vi "main_trackVideoFile.vi"() -> ()   [LabVIEW 2013]
uses:
  <vilib>/vision/Image Controls.llb/IMAQ Image.ctl
  <vilib>/vision/Avi.llb/IMAQ AVI2 Refnum.ctl
panel:
  out "Fitted Image":T1
  in  "SessionID":string
  in  "Exit program":bool
  in  "Start Session":bool
  in  "Tab Control":T2(tab)
  out "Eyetracker":T1(plugin-control)
  out "Pupil Radius":dbl[](graph)
  out "Avg freq":dbl caption="Eyetracker - Mean \nprocessing frequency (Hz)" format="%0.2f"
  in  "Save data to disk":bool
  out "Pupil marked":bool=TRUE
  out "Processed":T1(plugin-control)
  in  "Slowmo":bool=TRUE
  in  "Realtime":bool=TRUE
  in  "Fps to save images":u16(ring) items=["30", "60", "90", "120"]
  in  "Camera Fps":u16(ring) items=["30", "60", "90", "120"]
  in  "Look For (Threshold 2)":u32(ring)=1 items=["Bright Objects", "Dark Objects"]
  in  "Start / Stop Tracking":bool
  out "AVI Refnum - Eye":T3
  in  "Manual Threshold":cluster{sgl, sgl}(slide)={0.0, 150.0} caption="Threshold Range" scale=0.0..255.0
  in  "Pupiltracker Cam Connected":bool=TRUE
  out "Cropped Image":T1
  out "Processed Image":T1
  in  "Save folder":path=path "C:/Users/Eivind/Desktop"
  in  "Input video File":path=path "D:/RotationExperiments_v3_GCaMP6f+tdTomato/mouse013/session-m013-20161122-1807/labview_data/Block-11222016-1807-001-LightsON/EyeTracker-11222016-1807-001.avi"
  # "Optimize Tracking"
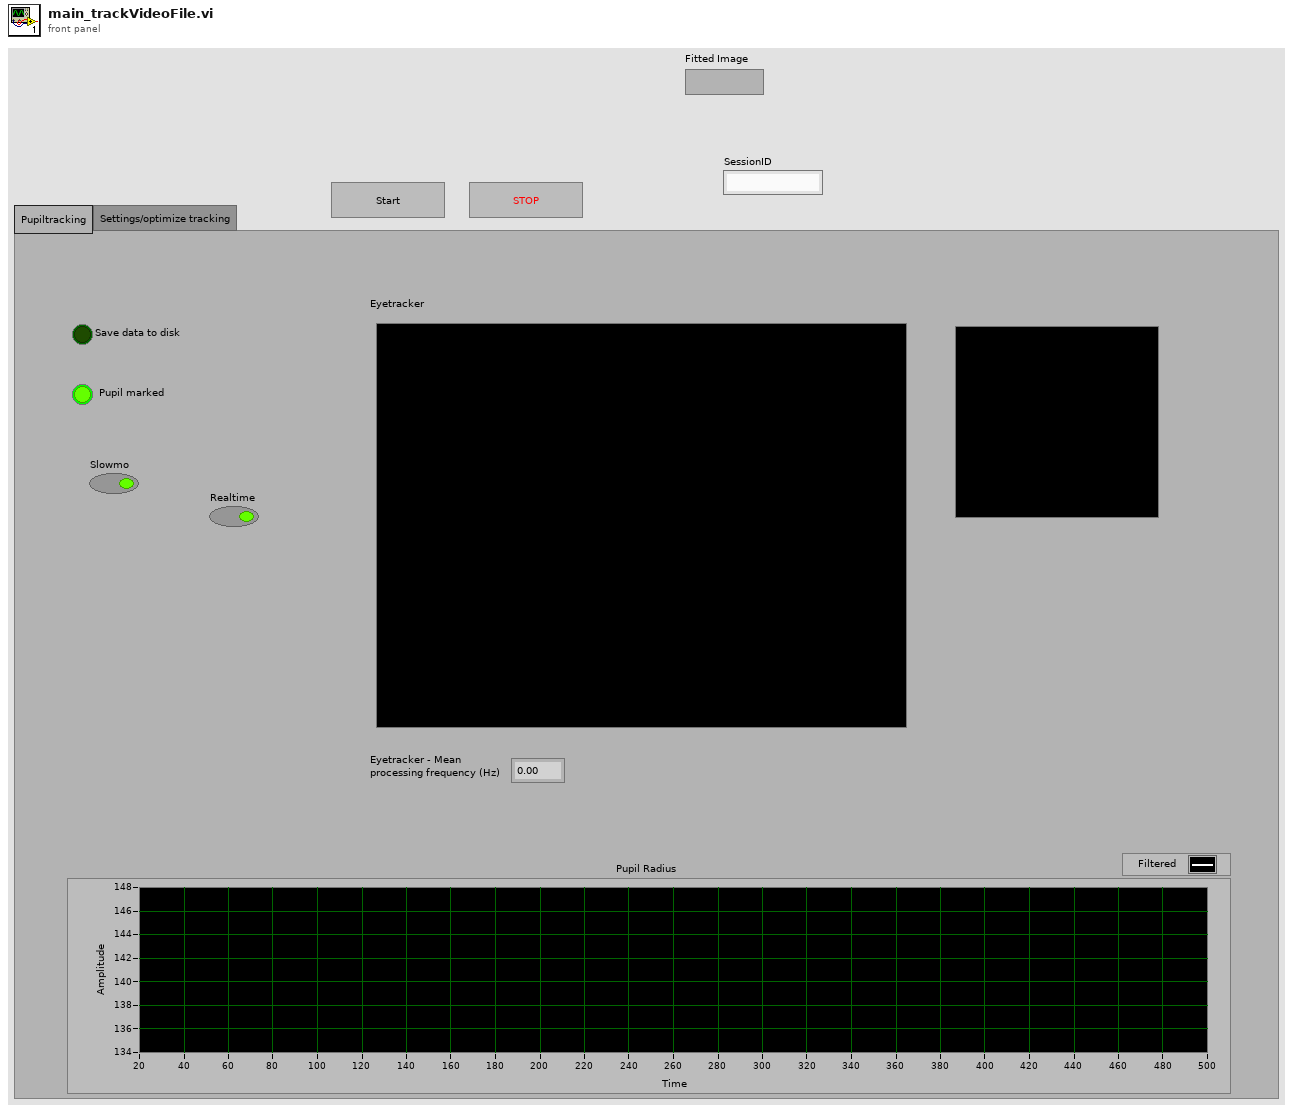
[diagram p1: front panel]
types:
  T1 = typedef "IMAQ Image.ctl" = refnum<image>
  T2 = enum32{"Pupiltracking", "Settings/optimize tracking"}
  T3 = typedef "IMAQ AVI2 Refnum.ctl" = refnum<k20>
  T4 = typedef "Image Type" = u32
  T5 = cluster{"Frame No":i32, "Circle time series":dbl[][], "Rectangle coordinates":i32[], "Annulus ROI":cluster{"ID":enum32{"External", "Internal"}, "Type":u32, i32[]}, "Annulus coordinates":i32[]}
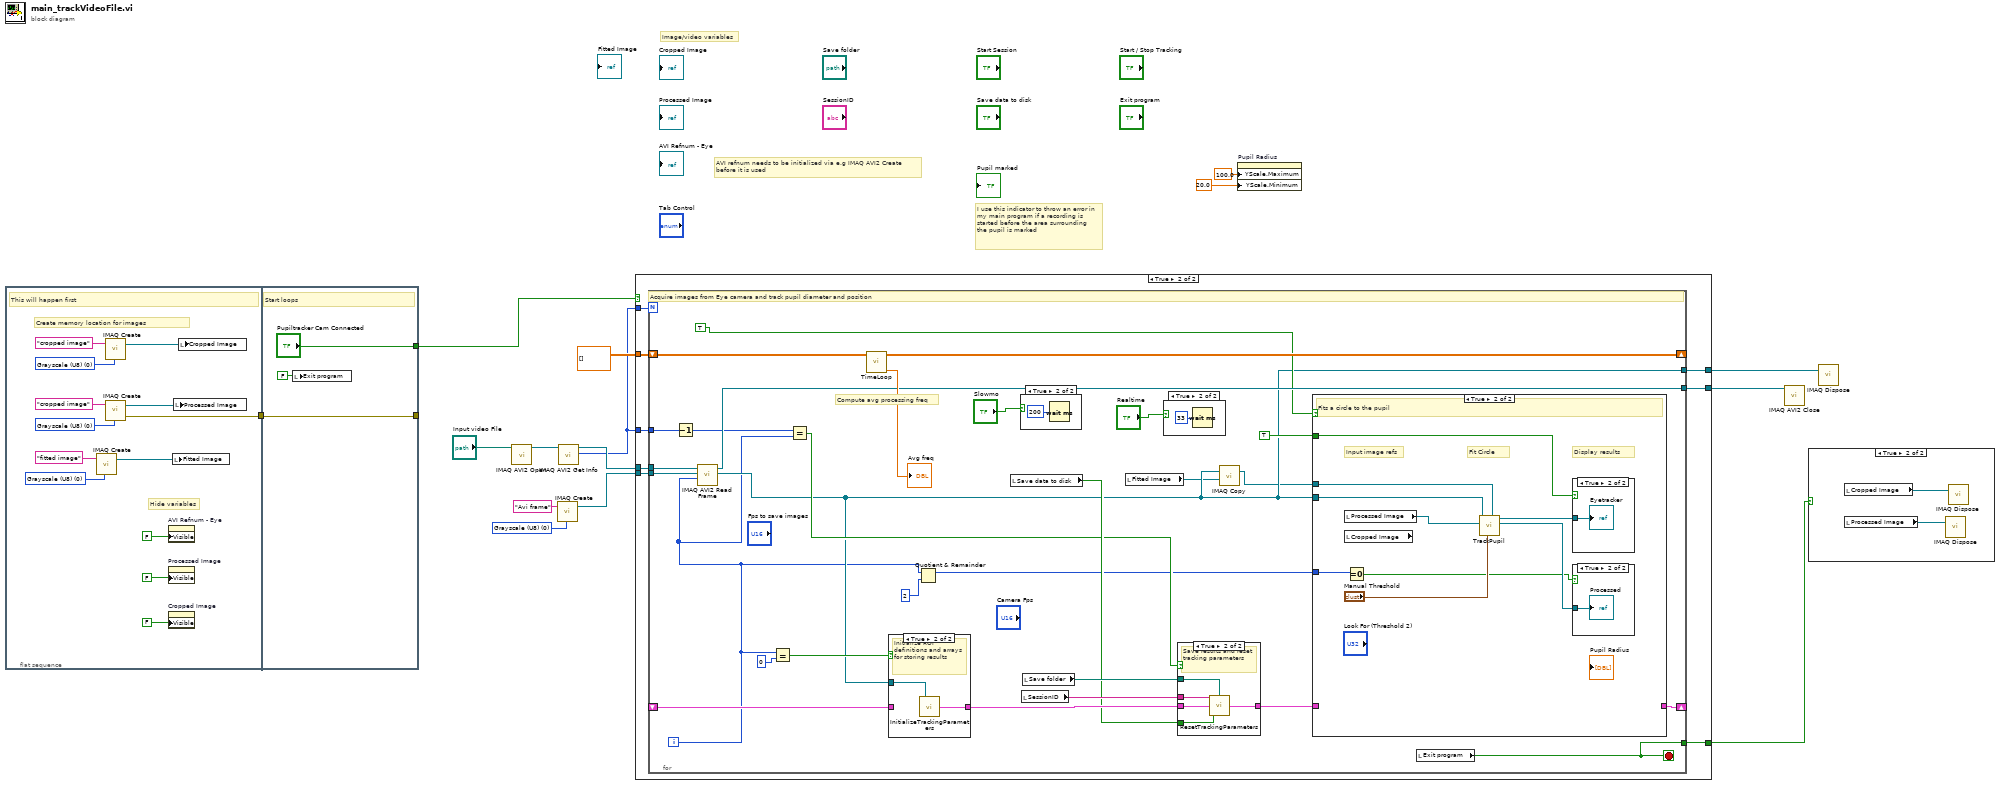
[diagram p0: block diagram]
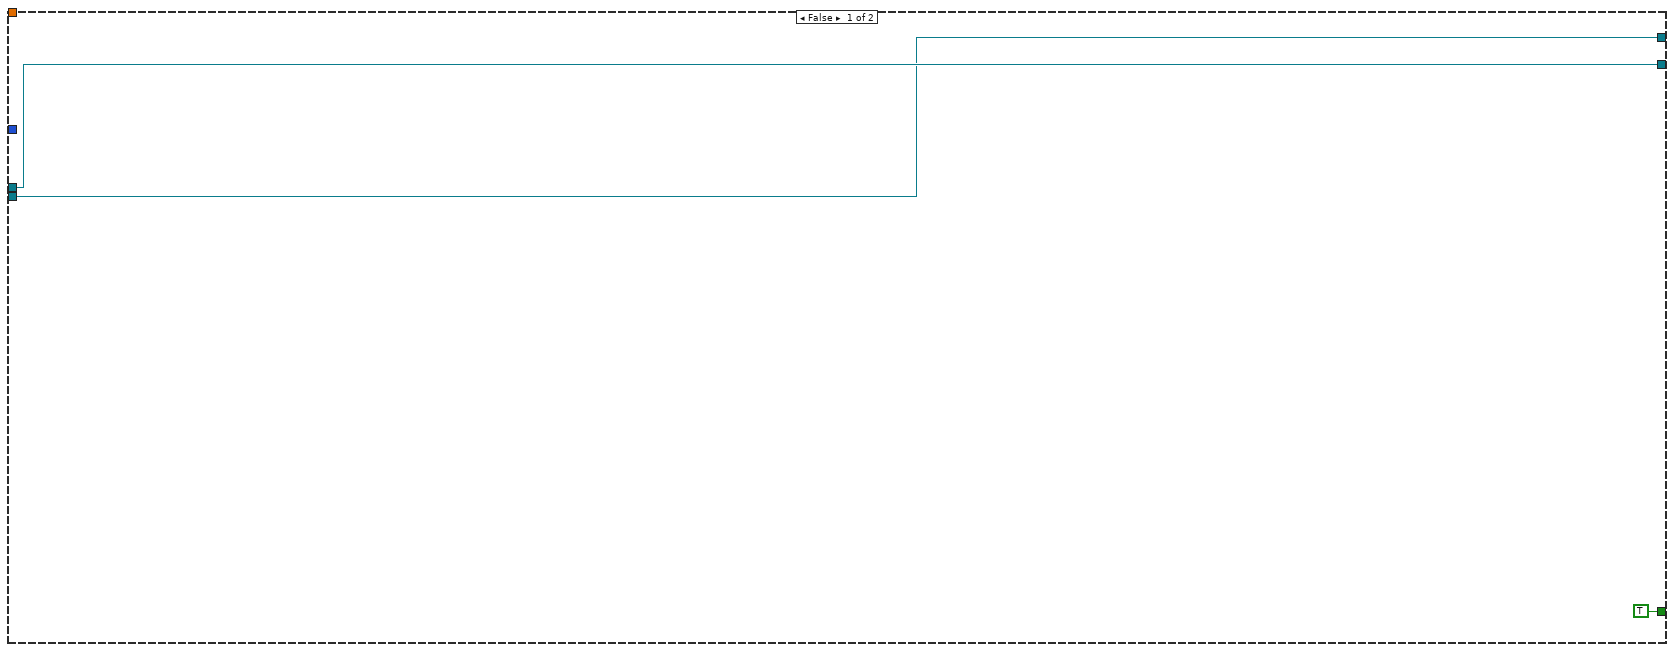
[diagram p3: hidden frame]
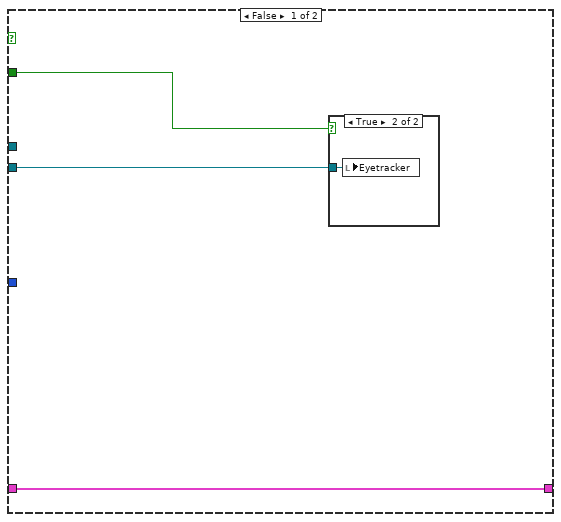
[diagram p8: hidden frame]
diagram:
  w8 = T4 0 items=["Grayscale (U8)", "Grayscale (I16)", "Grayscale (SGL)", "Complex (CSG)", "RGB (U32)", "HSL (U32)", "RGB (U64)", "Grayscale (U16)"] ("Image Type")
  # "AVI refnum needs to be initialized via e.g IMAQ AVI2 Create \nbefore it is used"
  # "I use this indicator to throw an error in my main program if a recording is started before the area surrounding the pupil is marked"
  # "Image/video variables"
  n1 = flat-sequence {
    tunnel: [w22] -> w14
    tunnel: [w31] -> _
    tunnel: w14 -> [w31]
    tunnel: ["Pupiltracker Cam Connected"] -> w13
    frame #0 {
      w17 = T4 0 items=["Grayscale (U8)", "Grayscale (I16)", "Grayscale (SGL)", "Complex (CSG)", "RGB (U32)", "HSL (U32)", "RGB (U64)", "Grayscale (U16)"] ("Image Type")
      w25 = T4 0 items=["Grayscale (U8)", "Grayscale (I16)", "Grayscale (SGL)", "Complex (CSG)", "RGB (U32)", "HSL (U32)", "RGB (U64)", "Grayscale (U16)"] ("Image Type")
      w28 = T4 0 items=["Grayscale (U8)", "Grayscale (I16)", "Grayscale (SGL)", "Complex (CSG)", "RGB (U32)", "HSL (U32)", "RGB (U64)", "Grayscale (U16)"] ("Image Type")
      # "Hide variables"
      # "Create memory location for images"
      # "This will happen first"
      n2 = call "IMAQ Create"("Image Name"="fitted image", "Image Type"=w17) -> ("New Image"=w16:T1)  [unwired: 3 in, 1 out]
      n3 = call "IMAQ Create"("Image Name"="cropped image", "Image Type"=w28) -> ("New Image"=w26:T1)  [unwired: 3 in, 1 out]
      n4 = call "IMAQ Create"("Image Name"="cropped image", "Image Type"=w25) -> ("New Image"=w23:T1, "error out"=w22:errorcluster)  [unwired: 3 in]
      n5 = property on="AVI Refnum - Eye" class="IMAQAVI (strict)"("Visible"=FALSE) -> ()  [unwired: 2 in, 2 out]
      n6 = property on="Processed Image" class="IMAQImage (strict)"("Visible"=FALSE) -> ()  [unwired: 2 in, 2 out]
      n7 = property on="Cropped Image" class="IMAQImage (strict)"("Visible"=FALSE) -> ()  [unwired: 2 in, 2 out]
      n8 = local write "Fitted Image"(w16) -> ()
      n9 = local write "Processed Image"(w23) -> ()
      n10 = local write "Cropped Image"(w26) -> ()
    }
    frame #1 {
      # "Start loops"
      n11 = local write "Exit program"(FALSE ("BtnExitLoops")) -> ()
    }
  }
  n12 = call "IMAQ AVI2 Open"("AVI File Path"="Input video File") -> ("AVI Refnum"=w10:T3)  [unwired: 9 in, 1 out]
  n13 = call "IMAQ Create"("Image Name"="Avi frame", "Image Type"=w8) -> ("New Image"=w7:T1)  [unwired: 3 in, 1 out]
  n14 = call "IMAQ AVI2 Get Info"("AVI Refnum"=w10) -> ("Number of Frames"=w3:u32, "AVI Refnum (duplicate)"=w6:T3)  [unwired: 6 in, 3 out]
  n15 = case shown="True" w13 {
    tunnel: dbl[][] [] -> [_ w42]
    tunnel: [TRUE ("Stopped") w36] -> w12
    tunnel: w7 -> [w32 w41]
    tunnel: w6 -> [w33 w40]
    tunnel: w3 -> [_ w39]
    tunnel: [w33 w38] -> w5
    tunnel: [w32 w37] -> w4
    tunnel: w3 -> [_ w35]
    frame False {
    }
    frame True {
      n16 = for {
        N: w39 -> [_]
        shift-right: [w71] -> _
        shift-left: w42 -> [w44]
        shift-right: [w67] -> _
        shift-left: _ -> [w66]
        tunnel: w41 -> [w62]
        tunnel: w40 -> [w61]
        tunnel: [w60] -> w38
        tunnel: [w53] -> w37
        tunnel: [w58] -> w36
        tunnel: w35 -> [w47]
        i -> [w43]
        stop <- w58 stop-if-true
        # "Compute avg processing freq"
        # "Acquire images from Eye camera and track pupil diameter and position"
        n17 = Decrement(x=w47) -> (x-1=w46:u32)
        n18 = call "IMAQ AVI2 Read Frame"("Frame Number"=w43, "Image"=w62, "AVI Refnum"=w61) -> ("Image Out"=w53:T1, "AVI Refnum (duplicate)"=w60:T3)  [unwired: 6 in, 1 out]
        n19 = Equal?(x=w43, y=0) -> (x = y?=w54:bool)
        n20 = Equal?(x=w46, y=w43) -> (x = y?=w57:bool)
        n21 = call "TimeLoop.vi"("Loop durations in"=w44) -> ("Average fps"=→"Avg freq":dbl, "Loop durations out"=w71:dbl[][])  [unwired: 5 in]
        n22 = case shown="True" w54 {
          tunnel: w53 -> [_ w82]
          tunnel: [w80 w81] -> w69
          tunnel: w66 -> [w80 _]
          frame False {
            # "Pass values"
          }
          frame True {
            # "Initialize ROI definitions and arrays for storing results"
            n23 = call "InitializeTrackingParameters.vi"("Refnum in"=w82) -> ("Circle fit parameters"=w81:T5)
          }
        }
        n24 = Quotient & Remainder(x=w43, y=2) -> (x-y*floor(x/y)=w49:i32)  [unwired: 1 out]
        n25 = local read "Save data to disk"() -> (w63:bool)
        n26 = case shown="True" "Slowmo" {
          frame False {
          }
          frame True {
            n27 = Wait (ms)(milliseconds to wait=u32 200) -> ()  [unwired: 1 out]
          }
        }
        n28 = local read "SessionID"() -> (w64:string)
        n29 = local read "Save folder"() -> (w65:path)
        n30 = local read "Fitted Image"() -> (w52:T1)
        n31 = case shown="True" "Realtime" {
          frame False {
          }
          frame True {
            n32 = Wait (ms)(milliseconds to wait=u32 33) -> ()  [unwired: 1 out]
          }
        }
        n33 = case shown="True" w57 {
          tunnel: w65 -> [_ w79]
          tunnel: w69 -> [w74 w78]
          tunnel: [w74 w77] -> w68
          tunnel: w63 -> [_ w76]
          tunnel: w64 -> [_ w75]
          frame False {
            # "Pass values"
          }
          frame True {
            # "Save results and reset tracking parameters"
            n34 = call "ResetTrackingParameters.vi"("file path"=w79, "Boolean"=w76, "Circle fit parameters in"=w78, "SessionID"=w75) -> ("Circle fit parameters out"=w77:T5)
          }
        }
        n35 = call "IMAQ Copy"("Image Dst"=w52, "Image Src"=w53) -> ("Image Dst Out"=w51:T1)  [unwired: 4 in, 1 out]
        n36 = case shown="True" TRUE ("x") {
          tunnel: w53 -> [w85 w90]
          tunnel: TRUE -> [w84 w93]
          tunnel: w68 -> [w83 _]
          tunnel: [w83 _] -> w67
          tunnel: w51 -> [_ w89]
          tunnel: w49 -> [_ w88]
          frame False {
            n37 = case shown="True" w84 {
              tunnel: w85 -> [_ w86]
              frame False {
              }
              frame True {
                n38 = local write "Eyetracker"(w86) -> ()
              }
            }
          }
          frame True {
            # "Input image refs"
            # "Display results"
            # "Fit Circle"
            # "Fits a circle to the pupil"
            n39 = local read "Processed Image"() -> (w91:T1)
            n40 = local read "Cropped Image"() -> ()  [unwired: 1 out]
            n41 = Equal To 0?(x=w88) -> (x = 0?=w87:bool)
            n42 = call "TrackPupil.vi"("Processed image"=w89, "Manual Threshold"="Manual Threshold", "Acquired image refnum"=w91, "Cropped image refnum"=w90) -> ("Processed image display refnum out"=w92:T1, "Fitted image refnum out"=w94:T1)  [unwired: 4 in, 2 out]
            n43 = case shown="True" w93 {
              tunnel: w94 -> [_ w96]
              frame False {
              }
              frame True {
                "Eyetracker" <- w96
              }
            }
            n44 = case shown="True" w87 {
              tunnel: w92 -> [_ w97]
              frame False {
              }
              frame True {
                "Processed" <- w97
              }
            }
          }
        }
        n45 = local read "Exit program"() -> (w58:bool)
      }
    }
  }
  n46 = property on="Pupil Radius" class="WFGraph (strict)"("YScale.Maximum"=100.0 ("Y Scale.Range:Maximum"), "YScale.Minimum"=20.0 ("Y Scale.Range:Minimum")) -> ()  [unwired: 2 in, 2 out]
  n47 = call "IMAQ AVI2 Close"("AVI Refnum"=w5) -> ()  [unwired: 10 in, 1 out]
  n48 = case shown="True" w12 {
    frame False {
    }
    frame True {
      n49 = local read "Cropped Image"() -> (w99:T1)
      n50 = local read "Processed Image"() -> (w98:T1)
      n51 = call "IMAQ Dispose"("Image"=w98) -> ()  [unwired: 5 in, 1 out]
      n52 = call "IMAQ Dispose"("Image"=w99) -> ()  [unwired: 5 in, 1 out]
    }
  }
  n53 = call "IMAQ Dispose"("Image"=w4) -> ()  [unwired: 5 in, 1 out]
